vi "NtfyLvFpga_SUB_ReadWriteConfigIni.vi"(6 "Read/Write(T)":bool, 8 "error in (no error)":errorcluster caption="エラー入力（エラーなし）", 9 "Config":T2={"SMTP Setting"={"smtp server"="", "From"="", "port number"=25, "userID"="", "password"="", "chk ssl"=FALSE, "chk server withSSL"=FALSE}, "SendTo"={"To 1"={"chk"=FALSE, "To"=""}, "To 2"={"chk"=FALSE, "To"=""}, "To 3"={"chk"=FALSE, "To"=""}}, "Prohibit time"={"chk enable"=FALSE, "start hour"=0, "end hour"=0}}, 11 "ConfigIni filepath":path=path "Config.ini") -> (0 "error out":errorcluster caption="エラー出力", 1 "Config out":T2={"SMTP Setting"={"smtp server"="", "From"="", "port number"=25, "userID"="", "password"="", "chk ssl"=FALSE, "chk server withSSL"=FALSE}, "SendTo"={"To 1"={"chk"=FALSE, "To"=""}, "To 2"={"chk"=FALSE, "To"=""}, "To 3"={"chk"=FALSE, "To"=""}}, "Prohibit time"={"chk enable"=FALSE, "start hour"=0, "end hour"=0}})   [LabVIEW 2013]
uses:
  NtfyLvFpga_Typedef_SMTPSetting.ctl
  <vilib>/Utility/config.llb/Write Key (String).vi
  <vilib>/Utility/config.llb/Write Key (I32).vi
  <vilib>/Utility/config.llb/Write Key (Boolean).vi
  <vilib>/Utility/config.llb/Read Key (String).vi
  <vilib>/Utility/config.llb/Read Key (I32).vi
  <vilib>/Utility/config.llb/Read Key (Boolean).vi
  <vilib>/Utility/config.llb/NI_LVConfig.lvlib
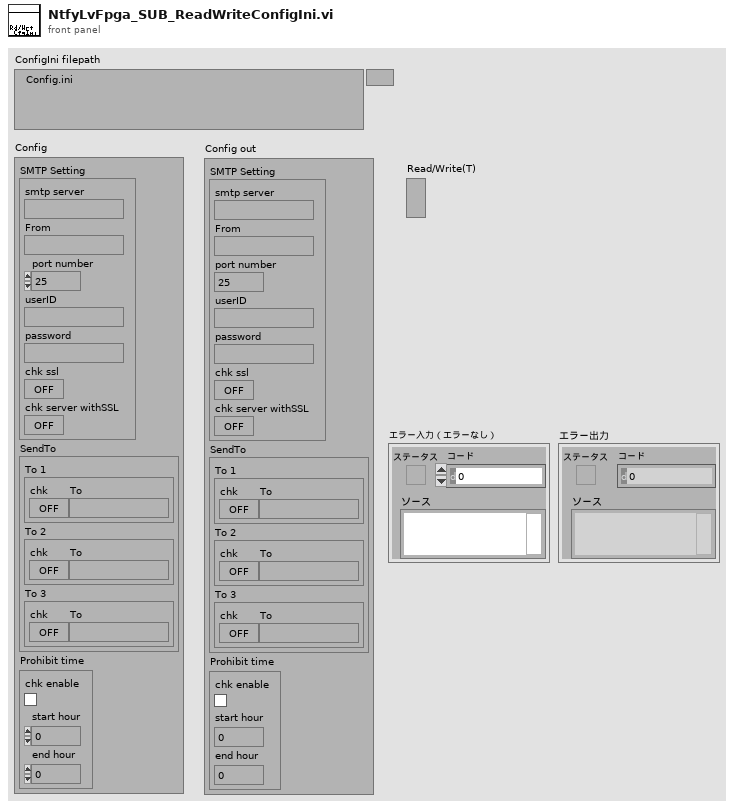
[diagram p1: front panel]
types:
  T1 = typedef "NtfyLvFpga_Typedef_SMTPSetting.ctl" = cluster{"smtp server":string, "From":string, "port number":i32, "userID":string, "password":string, "chk ssl":bool, "chk server withSSL":bool}
  T2 = cluster{"SMTP Setting":T1, "SendTo":cluster{"To 1":cluster{"chk":bool, "To":string}, "To 2":cluster{"chk":bool, "To":string}, "To 3":cluster{"chk":bool, "To":string}}, "Prohibit time":cluster{"chk enable":bool, "start hour":u8, "end hour":u8}}
  T3 = cluster{"To 1":cluster{"chk":bool, "To":string}, "To 2":cluster{"chk":bool, "To":string}, "To 3":cluster{"chk":bool, "To":string}}
  T4 = cluster{"chk enable":bool, "start hour":u8, "end hour":u8}
  T5 = typedef "NI_LVConfig.lvlib/Config Data RefNum.ctl" = refnum<k1>
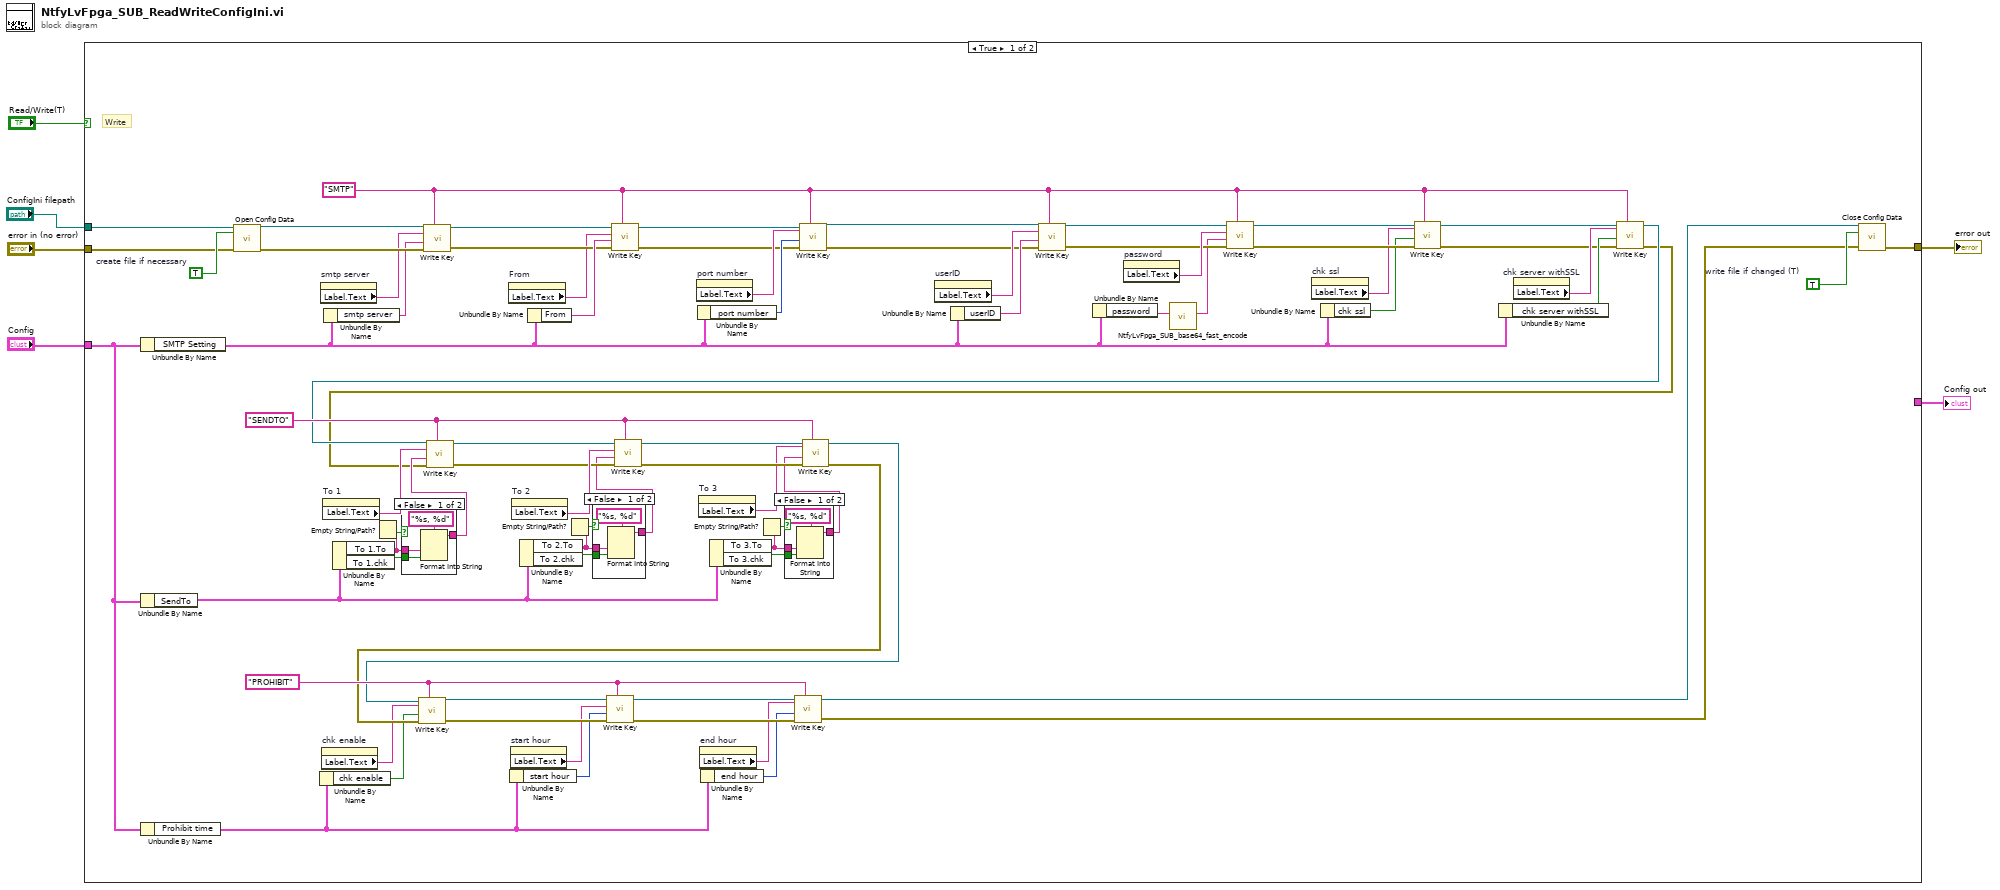
[diagram p0: block diagram]
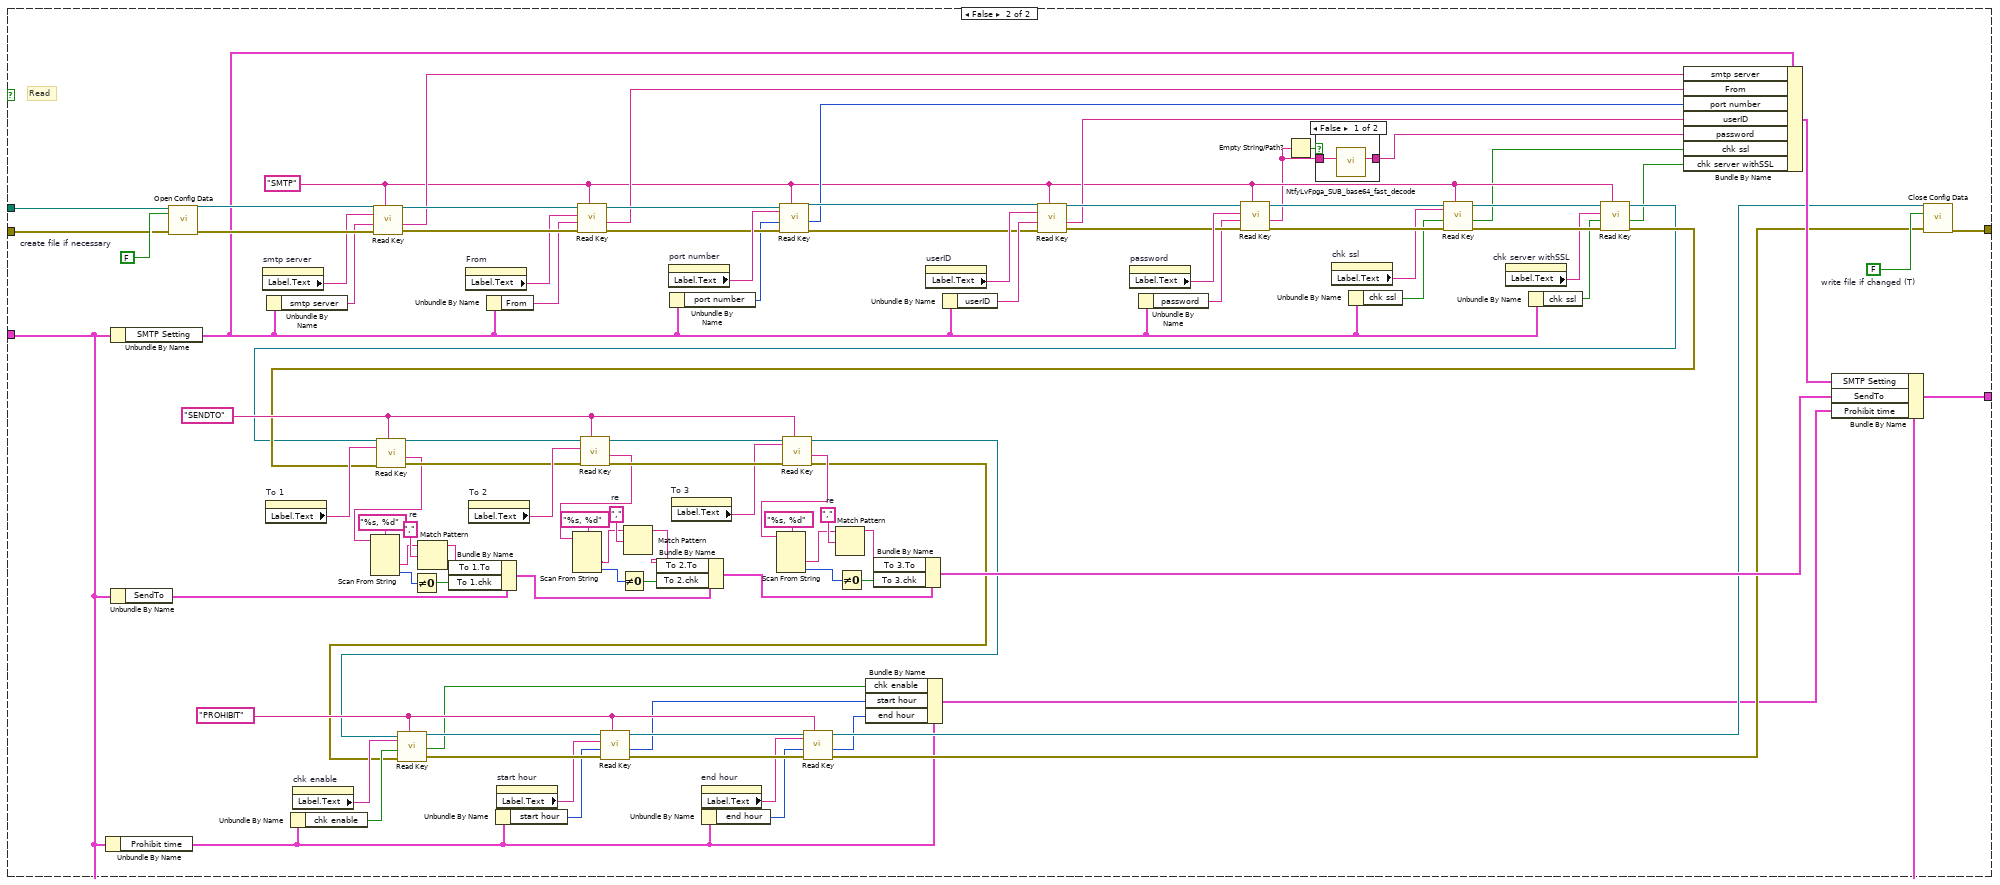
[diagram p5: hidden frame]
diagram:
  n1 = case shown="TRUE" "Read/Write(T)" {
    tunnel: "error in (no error)" -> [w81 w195]
    tunnel: [w79 w193] -> w5
    tunnel: "ConfigIni filepath" -> [w80 w194]
    tunnel: "Config" -> [w22 w109]
    tunnel: [_ w140] -> w1
    frame True {
      w23 = "PROHIBIT"
      w49 = "SENDTO"
      w35 = "SMTP"
      w78 = TRUE  # write file if changed (T)
      w82 = TRUE  # create file if necessary
      # "Write"
      n2 = Unbundle By Name(w22) -> ("SMTP Setting"=w8:T1)
      n3 = Unbundle By Name(w22) -> ("SendTo"=w42:T3)
      n4 = Unbundle By Name(w22) -> ("Prohibit time"=w17:T4)
      n5 = call <vilib>:"Open Config Data.vi"("error in (no error)"=w81, "create file if necessary (T)"=w82, "configuration file path"=w80) -> ("error out"=w76:errorcluster, "refnum"=w77:T5)  [unwired: 6 in, 1 out]
      n6 = Unbundle By Name(w17) -> ("chk enable"=w16:bool)
      n7 = property on="smtp server" class="Str"() -> ("Label.Text"=w74:string)  [unwired: 2 in, 2 out]
      n8 = property on="chk enable" class="Bool （指定）"() -> ("Label.Text"=w13:string)  [unwired: 2 in, 2 out]
      n9 = property on="To 1" class="Clust （指定）"() -> ("Label.Text"=w50:string)  [unwired: 2 in, 2 out]
      n10 = Unbundle By Name(w8) -> ("smtp server"=w75:string)
      n11 = Unbundle By Name(w42) -> ("To 1.To"=w34:string, "To 1.chk"=w48:bool)
      n12 = Empty String/Path?(string/path=w34) -> (empty?=w33:bool)
      n13 = case shown="FALSE" w33 {
        tunnel: w34 -> [w93 _]
        tunnel: w48 -> [w92 _]
        tunnel: [w91 _] -> w47
        frame False {
          n14 = Format Into String(format string="%s, %d", w93, w92) -> (resulting string=w91:string)  [unwired: 2 in, 1 out]
        }
        frame True {
        }
      }
      n15 = call-poly <vilib>:"Write Key.vi"("section"=w35, "error in (no error)"=w76, "value"=w75, "key"=w74, "refnum"=w77) -> ("error out"=w70:errorcluster, "refnum out"=w67:T5)  [unwired: 4 in, 1 out]
      n16 = property on="From" class="Str"() -> ("Label.Text"=w68:string)  [unwired: 2 in, 2 out]
      n17 = Unbundle By Name(w17) -> ("start hour"=w15:u8)
      n18 = property on="start hour" class="DigNum （指定）"() -> ("Label.Text"=w12:string)  [unwired: 2 in, 2 out]
      n19 = property on="To 2" class="Clust （指定）"() -> ("Label.Text"=w54:string)  [unwired: 2 in, 2 out]
      n20 = Unbundle By Name(w42) -> ("To 2.To"=w32:string, "To 2.chk"=w46:bool)
      n21 = Unbundle By Name(w8) -> ("From"=w73:string)
      n22 = Empty String/Path?(string/path=w32) -> (empty?=w31:bool)
      n23 = case shown="FALSE" w31 {
        tunnel: w46 -> [w90 _]
        tunnel: w32 -> [w89 _]
        tunnel: [w87 _] -> w44
        frame False {
          n24 = Format Into String(format string="%s, %d", w89, w90) -> (resulting string=w87:string)  [unwired: 2 in, 1 out]
        }
        frame True {
        }
      }
      n25 = call-poly <vilib>:"Write Key.vi"("section"=w35, "error in (no error)"=w70, "value"=w73, "key"=w68, "refnum"=w67) -> ("error out"=w69:errorcluster, "refnum out"=w66:T5)  [unwired: 4 in, 1 out]
      n26 = property on="port number" class="DigNum （指定）"() -> ("Label.Text"=w71:string)  [unwired: 2 in, 2 out]
      n27 = Unbundle By Name(w8) -> ("port number"=w72:i32)
      n28 = property on="To 3" class="Clust （指定）"() -> ("Label.Text"=w51:string)  [unwired: 2 in, 2 out]
      n29 = property on="end hour" class="DigNum （指定）"() -> ("Label.Text"=w11:string)  [unwired: 2 in, 2 out]
      n30 = Unbundle By Name(w17) -> ("end hour"=w14:u8)
      n31 = Unbundle By Name(w42) -> ("To 3.To"=w29:string, "To 3.chk"=w45:bool)
      n32 = Empty String/Path?(string/path=w29) -> (empty?=w30:bool)
      n33 = case shown="FALSE" w30 {
        tunnel: w29 -> [w85 _]
        tunnel: w45 -> [w84 _]
        tunnel: [w83 _] -> w43
        frame False {
          n34 = Format Into String(format string="%s, %d", w85, w84) -> (resulting string=w83:string)  [unwired: 2 in, 1 out]
        }
        frame True {
        }
      }
      n35 = call-poly <vilib>:"Write Key.vi"("section"=w35, "error in (no error)"=w69, "value"=w72, "key"=w71, "refnum"=w66) -> ("error out"=w57:errorcluster, "refnum out"=w58:T5)  [unwired: 4 in, 1 out]
      n36 = property on="userID" class="Str"() -> ("Label.Text"=w60:string)  [unwired: 2 in, 2 out]
      n37 = Unbundle By Name(w8) -> ("userID"=w59:string)
      n38 = call-poly <vilib>:"Write Key.vi"("section"=w35, "error in (no error)"=w57, "value"=w59, "key"=w60, "refnum"=w58) -> ("error out"=w10:errorcluster, "refnum out"=w64:T5)  [unwired: 4 in, 1 out]
      n39 = Unbundle By Name(w8) -> ("password"=w28:string)
      n40 = property on="password" class="Str"() -> ("Label.Text"=w63:string)  [unwired: 2 in, 2 out]
      n41 = call "NtfyLvFpga_SUB_base64_fast_encode.vi"("string in (not encoded)"=w28) -> ("string out (base64-encoded)"=w9:string)  [unwired: 9 in, 1 out]
      n42 = call-poly <vilib>:"Write Key.vi"("section"=w35, "error in (no error)"=w10, "value"=w9, "key"=w63, "refnum"=w64) -> ("error out"=w62:errorcluster, "refnum out"=w65:T5)  [unwired: 4 in, 1 out]
      n43 = property on="chk ssl" class="Bool （指定）"() -> ("Label.Text"=w61:string)  [unwired: 2 in, 2 out]
      n44 = Unbundle By Name(w8) -> ("chk ssl"=w7:bool)
      n45 = call-poly <vilib>:"Write Key.vi"("section"=w35, "error in (no error)"=w62, "value"=w7, "key"=w61, "refnum"=w65) -> ("error out"=w36:errorcluster, "refnum out"=w37:T5)  [unwired: 4 in, 1 out]
      n46 = Unbundle By Name(w8) -> ("chk server withSSL"=w41:bool)
      n47 = property on="chk server withSSL" class="Bool （指定）"() -> ("Label.Text"=w40:string)  [unwired: 2 in, 2 out]
      n48 = call-poly <vilib>:"Write Key.vi"("section"=w35, "error in (no error)"=w36, "value"=w41, "key"=w40, "refnum"=w37) -> ("error out"=w38:errorcluster, "refnum out"=w39:T5)  [unwired: 4 in, 1 out]
      n49 = call-poly <vilib>:"Write Key.vi"("section"=w49, "error in (no error)"=w38, "value"=w47, "key"=w50, "refnum"=w39) -> ("error out"=w52:errorcluster, "refnum out"=w55:T5)  [unwired: 4 in, 1 out]
      n50 = call-poly <vilib>:"Write Key.vi"("section"=w49, "error in (no error)"=w52, "value"=w44, "key"=w54, "refnum"=w55) -> ("error out"=w53:errorcluster, "refnum out"=w56:T5)  [unwired: 4 in, 1 out]
      n51 = call-poly <vilib>:"Write Key.vi"("section"=w49, "error in (no error)"=w53, "value"=w43, "key"=w51, "refnum"=w56) -> ("error out"=w18:errorcluster, "refnum out"=w19:T5)  [unwired: 4 in, 1 out]
      n52 = call-poly <vilib>:"Write Key.vi"("section"=w23, "error in (no error)"=w18, "value"=w16, "key"=w13, "refnum"=w19) -> ("error out"=w27:errorcluster, "refnum out"=w25:T5)  [unwired: 4 in, 1 out]
      n53 = call-poly <vilib>:"Write Key.vi"("section"=w23, "error in (no error)"=w27, "value"=w15, "key"=w12, "refnum"=w25) -> ("error out"=w26:errorcluster, "refnum out"=w24:T5)  [unwired: 4 in, 1 out]
      n54 = call-poly <vilib>:"Write Key.vi"("section"=w23, "error in (no error)"=w26, "value"=w14, "key"=w11, "refnum"=w24) -> ("error out"=w20:errorcluster, "refnum out"=w21:T5)  [unwired: 4 in, 1 out]
      n55 = call <vilib>:"Close Config Data.vi"("error in (no error)"=w20, "write file if changed (T)"=w78, "refnum"=w21) -> ("error out"=w79:errorcluster)  [unwired: 7 in, 1 out]
    }
    frame False {
      w114 = "PROHIBIT"
      w124 = ","  # re
      w125 = ","  # re
      w128 = ","  # re
      w165 = "SENDTO"
      w130 = "SMTP"
      w192 = FALSE  # write file if changed (T)
      w196 = FALSE  # create file if necessary
      # "Read"
      n56 = Unbundle By Name(w109) -> ("Prohibit time"=w102:T4)
      n57 = Unbundle By Name(w109) -> ("SMTP Setting"=w133:T1)
      n58 = Unbundle By Name(w109) -> ("SendTo"=w152:T3)
      n59 = call <vilib>:"Open Config Data.vi"("error in (no error)"=w195, "create file if necessary (T)"=w196, "configuration file path"=w194) -> ("error out"=w190:errorcluster, "refnum"=w191:T5)  [unwired: 6 in, 1 out]
      n60 = property on="smtp server" class="Str"() -> ("Label.Text"=w189:string)  [unwired: 2 in, 2 out]
      n61 = property on="To 1" class="Clust （指定）"() -> ("Label.Text"=w166:string)  [unwired: 2 in, 2 out]
      n62 = Unbundle By Name(w133) -> ("smtp server"=w161:string)
      n63 = Unbundle By Name(w102) -> ("chk enable"=w113:bool)
      n64 = property on="chk enable" class="Bool （指定）"() -> ("Label.Text"=w112:string)  [unwired: 2 in, 2 out]
      n65 = call-poly <vilib>:"Read Key.vi"("section"=w130, "error in (no error)"=w190, "default value"=w161, "key"=w189, "refnum"=w191) -> ("error out"=w187:errorcluster, "value"=w154:string, "refnum out"=w184:T5)  [unwired: 3 in, 1 out]
      n66 = property on="From" class="Str"() -> ("Label.Text"=w185:string)  [unwired: 2 in, 2 out]
      n67 = property on="To 2" class="Clust （指定）"() -> ("Label.Text"=w170:string)  [unwired: 2 in, 2 out]
      n68 = Unbundle By Name(w133) -> ("From"=w160:string)
      n69 = Unbundle By Name(w102) -> ("start hour"=w103:u8)
      n70 = property on="start hour" class="DigNum （指定）"() -> ("Label.Text"=w111:string)  [unwired: 2 in, 2 out]
      n71 = call-poly <vilib>:"Read Key.vi"("section"=w130, "error in (no error)"=w187, "default value"=w160, "key"=w185, "refnum"=w184) -> ("error out"=w186:errorcluster, "value"=w153:string, "refnum out"=w183:T5)  [unwired: 3 in, 1 out]
      n72 = property on="port number" class="DigNum （指定）"() -> ("Label.Text"=w188:string)  [unwired: 2 in, 2 out]
      n73 = Unbundle By Name(w133) -> ("port number"=w159:i32)
      n74 = property on="To 3" class="Clust （指定）"() -> ("Label.Text"=w167:string)  [unwired: 2 in, 2 out]
      n75 = property on="end hour" class="DigNum （指定）"() -> ("Label.Text"=w110:string)  [unwired: 2 in, 2 out]
      n76 = Unbundle By Name(w102) -> ("end hour"=w104:u8)
      n77 = call-poly <vilib>:"Read Key.vi"("section"=w130, "error in (no error)"=w186, "default value"=w159, "key"=w188, "refnum"=w183) -> ("error out"=w173:errorcluster, "value"=w155:i32, "refnum out"=w174:T5)  [unwired: 3 in, 1 out]
      n78 = property on="userID" class="Str"() -> ("Label.Text"=w176:string)  [unwired: 2 in, 2 out]
      n79 = Unbundle By Name(w133) -> ("userID"=w175:string)
      n80 = call-poly <vilib>:"Read Key.vi"("section"=w130, "error in (no error)"=w173, "default value"=w175, "key"=w176, "refnum"=w174) -> ("error out"=w178:errorcluster, "value"=w156:string, "refnum out"=w181:T5)  [unwired: 3 in, 1 out]
      n81 = property on="password" class="Str"() -> ("Label.Text"=w180:string)  [unwired: 2 in, 2 out]
      n82 = Unbundle By Name(w133) -> ("password"=w157:string)
      n83 = call-poly <vilib>:"Read Key.vi"("section"=w130, "error in (no error)"=w178, "default value"=w157, "key"=w180, "refnum"=w181) -> ("error out"=w179:errorcluster, "value"=w97:string, "refnum out"=w182:T5)  [unwired: 3 in, 1 out]
      n84 = Empty String/Path?(string/path=w97) -> (empty?=w119:bool)
      n85 = case shown="FALSE" w119 {
        tunnel: w97 -> [w198 w199]
        tunnel: [w197 w199] -> w96
        frame False {
          n86 = call "NtfyLvFpga_SUB_base64_fast_decode.vi"("string in (base64-encoded)"=w198) -> ("string out (decoded)"=w197:string)  [unwired: 9 in, 1 out]
        }
        frame True {
        }
      }
      n87 = property on="chk ssl" class="Bool （指定）"() -> ("Label.Text"=w177:string)  [unwired: 2 in, 2 out]
      n88 = Unbundle By Name(w133) -> ("chk ssl"=w158:bool)
      n89 = call-poly <vilib>:"Read Key.vi"("section"=w130, "error in (no error)"=w179, "default value"=w158, "key"=w177, "refnum"=w182) -> ("error out"=w137:errorcluster, "value"=w95:bool, "refnum out"=w138:T5)  [unwired: 3 in, 1 out]
      n90 = property on="chk server withSSL" class="Bool （指定）"() -> ("Label.Text"=w134:string)  [unwired: 2 in, 2 out]
      n91 = Unbundle By Name(w133) -> ("chk ssl"=w132:bool)
      n92 = call-poly <vilib>:"Read Key.vi"("section"=w130, "error in (no error)"=w137, "default value"=w132, "key"=w134, "refnum"=w138) -> ("error out"=w136:errorcluster, "value"=w131:bool, "refnum out"=w135:T5)  [unwired: 3 in, 1 out]
      n93 = call-poly <vilib>:"Read Key.vi"("section"=w165, "error in (no error)"=w136, "key"=w166, "refnum"=w135) -> ("error out"=w168:errorcluster, "value"=w150:string, "refnum out"=w171:T5)  [unwired: 4 in, 1 out]
      n94 = Scan From String(format string="%s, %d", input string=w150) -> (output 1=w127:string, output 2=w151:i32)  [unwired: 4 in, 3 out]
      n95 = Not Equal To 0?(x=w151) -> (x != 0?=w149:bool)
      n96 = Match Pattern(string=w127, regular expression=w128) -> (before substring=w126:string)  [unwired: 1 in, 3 out]
      n97 = Bundle By Name(cluster=w152, "To 1.To"=w126, "To 1.chk"=w149) -> (w146:T3)
      n98 = call-poly <vilib>:"Read Key.vi"("section"=w165, "error in (no error)"=w168, "key"=w170, "refnum"=w171) -> ("error out"=w169:errorcluster, "value"=w147:string, "refnum out"=w172:T5)  [unwired: 4 in, 1 out]
      n99 = Scan From String(format string="%s, %d", input string=w147) -> (output 1=w121:string, output 2=w145:i32)  [unwired: 4 in, 3 out]
      n100 = Not Equal To 0?(x=w145) -> (x != 0?=w148:bool)
      n101 = Match Pattern(string=w121, regular expression=w125) -> (before substring=w120:string)  [unwired: 1 in, 3 out]
      n102 = Bundle By Name(cluster=w146, "To 2.To"=w120, "To 2.chk"=w148) -> (w129:T3)
      n103 = call-poly <vilib>:"Read Key.vi"("section"=w165, "error in (no error)"=w169, "key"=w167, "refnum"=w172) -> ("error out"=w105:errorcluster, "value"=w143:string, "refnum out"=w106:T5)  [unwired: 4 in, 1 out]
      n104 = call-poly <vilib>:"Read Key.vi"("section"=w114, "error in (no error)"=w105, "default value"=w113, "key"=w112, "refnum"=w106) -> ("error out"=w118:errorcluster, "value"=w101:bool, "refnum out"=w116:T5)  [unwired: 3 in, 1 out]
      n105 = call-poly <vilib>:"Read Key.vi"("section"=w114, "error in (no error)"=w118, "default value"=w103, "key"=w111, "refnum"=w116) -> ("error out"=w117:errorcluster, "value"=w100:i32, "refnum out"=w115:T5)  [unwired: 3 in, 1 out]
      n106 = Scan From String(format string="%s, %d", input string=w143) -> (output 1=w123:string, output 2=w142:i32)  [unwired: 4 in, 3 out]
      n107 = call-poly <vilib>:"Read Key.vi"("section"=w114, "error in (no error)"=w117, "default value"=w104, "key"=w110, "refnum"=w115) -> ("error out"=w107:errorcluster, "value"=w99:i32, "refnum out"=w108:T5)  [unwired: 3 in, 1 out]
      n108 = Match Pattern(string=w123, regular expression=w124) -> (before substring=w122:string)  [unwired: 1 in, 3 out]
      n109 = Not Equal To 0?(x=w142) -> (x != 0?=w144:bool)
      n110 = Bundle By Name(cluster=w102, "chk enable"=w101, "start hour"=w100, "end hour"=w99) -> (w98:T4)
      n111 = Bundle By Name(cluster=w129, "To 3.To"=w122, "To 3.chk"=w144) -> (w139:T3)
      n112 = Bundle By Name(cluster=w133, "smtp server"=w154, "From"=w153, "port number"=w155, "userID"=w156, "password"=w96, "chk ssl"=w95, "chk server withSSL"=w131) -> (w141:T1)
      n113 = Bundle By Name(cluster=w109, "SMTP Setting"=w141, "SendTo"=w139, "Prohibit time"=w98) -> (w140:T2)
      n114 = call <vilib>:"Close Config Data.vi"("error in (no error)"=w107, "write file if changed (T)"=w192, "refnum"=w108) -> ("error out"=w193:errorcluster)  [unwired: 7 in, 1 out]
    }
  }
  "error out" <- w5
  "Config out" <- w1
